vi "Spectrometer Triax 550 (N.O.).vi"(7 "Force Reset? (F)":bool, 8 "error in (no error)":errorcluster, 10 "Ref to a Status Box":refnum<vi>, 11 "Cluster In":T4) -> (0 "error out":errorcluster, 3 "Cluster Out":T4)   [LabVIEW 2009]
uses:
  JY-SPEX-TRIAX/controls.llb/Monochromator System Number.ctl
  JY-SPEX-TRIAX/controls.llb/Mirror Position.ctl
  JY-SPEX-TRIAX/controls.llb/Turret Position (TRIAX).ctl
  Global/GPIB Numbers.vi
  JY-SPEX-TRIAX/JY-SPEX-TRIAX.lvlib
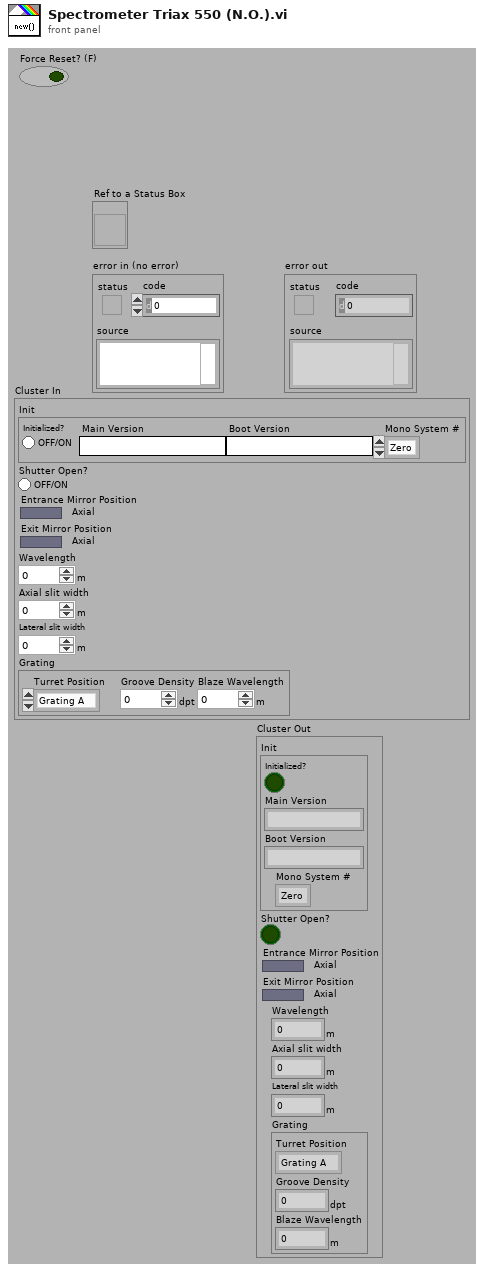
[diagram p1: front panel]
types:
  T1 = typedef "JY-SPEX-TRIAX.lvlib/Monochromator System Number.ctl" = enum16{"Zero", "One"}
  T2 = typedef "JY-SPEX-TRIAX.lvlib/Mirror Position.ctl" = bool
  T3 = typedef "JY-SPEX-TRIAX.lvlib/Turret Position (TRIAX).ctl" = enum16{"Grating A", "Grating B", "Grating C"}
  T4 = cluster{"Init":cluster{"Initialized?":bool, "Main Version":string, "Boot Version":string, "Mono System #":T1}, "Shutter Open?":bool, "Entrance Mirror Position":T2, "Exit Mirror Position":T2, "Wavelength":dbl[unit], "Axial slit width":dbl[unit], "Lateral slit width":dbl[unit], "Grating":cluster{"Turret Position":T3, "Groove Density":dbl[unit], "Blaze Wavelength":dbl[unit]}}
  T5 = typedef "GPIB Type Def.ctl" = cluster{"Name":string, "bus":dbl, "GPIB":dbl, "GPIB as string":string, "byte":i32, "VISA Resource Name":refnum<visa-resource-name>}
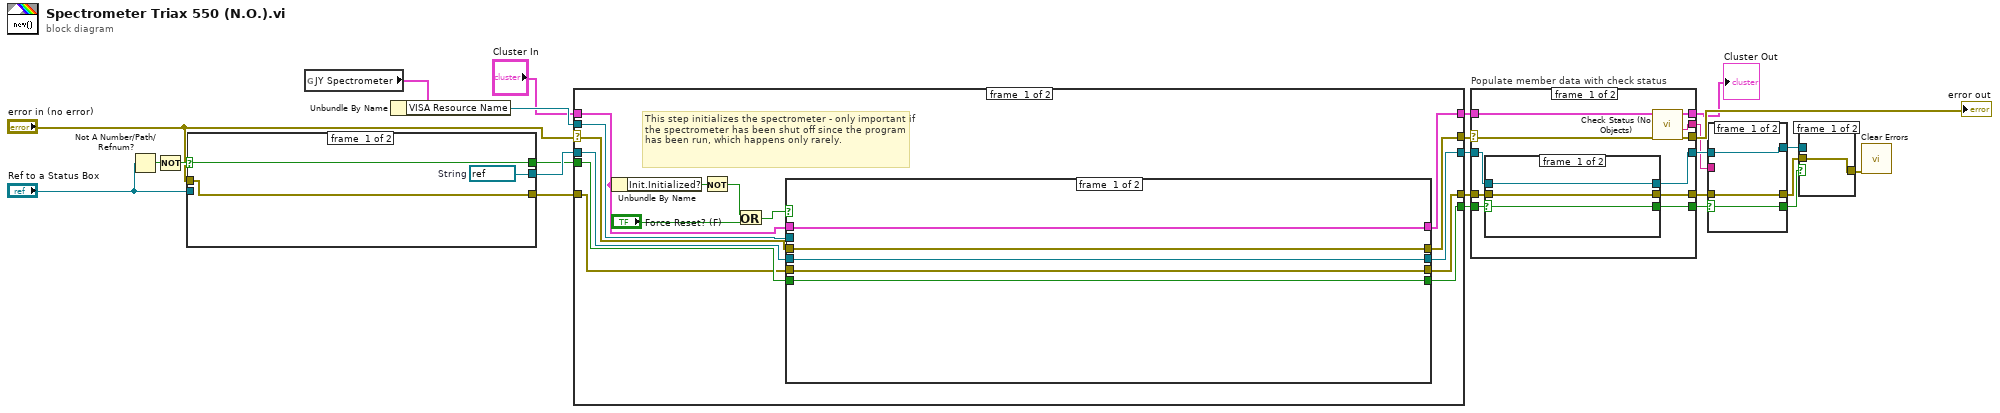
[diagram p0: block diagram]
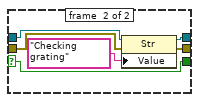
[diagram p2: hidden frame]
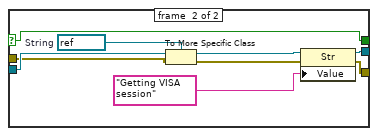
[diagram p4: hidden frame]
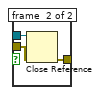
[diagram p5: hidden frame]
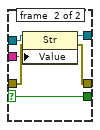
[diagram p6: hidden frame]
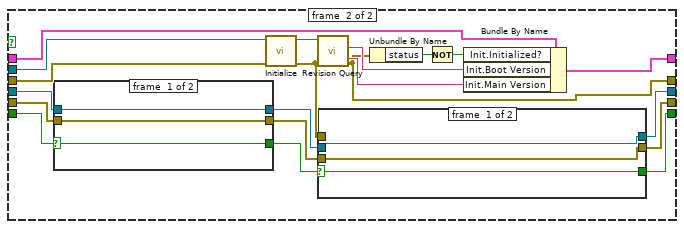
[diagram p7: hidden frame]
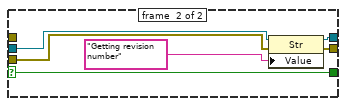
[diagram p8: hidden frame]
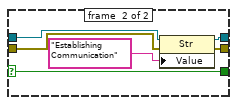
[diagram p9: hidden frame]
diagram:
  n1 = Not A Number/Path/Refnum?(number/path/refnum="Ref to a Status Box") -> (NaN/Path/Refnum?=w19:bool)
  n2 = Not(x=w19) -> (.not. x?=w7:bool)
  n3 = case shown="True" w7 {
    selector: w7 -> [w27 w34]
    tunnel: "error in (no error)" -> [w28 w29]
    tunnel: [w28 w37] -> w23
    tunnel: "Ref to a Status Box" -> [_ w32]
    tunnel: [w26 w35] -> w25
    tunnel: [w27 w34] -> w24
    frame #0 {
      w26 = refnum<vi> refnum  # String
    }
    frame #1 {
      w33 = refnum<vi> refnum  # String
      n4 = To More Specific Class(target class=w33, reference=w32, error in=w29) -> (specific class reference=w30:refnum<vi>, error out=w31:errorcluster)
      n5 = property class="Str"(reference=w30, error in=w31, "Value"="Getting VISA session") -> (reference out=w35:refnum<vi>, error out=w37:errorcluster)
    }
  }
  n6 = global read "GPIB Numbers.vi" "JY Spectrometer"() -> (w5:T5)
  n7 = Unbundle By Name(w5) -> ("VISA Resource Name"=w3:refnum<visa-resource-name>)
  n8 = case shown="No Error" "error in (no error)" {
    selector: "error in (no error)" -> [w43 w100]
    tunnel: [w46 w100] -> w6
    tunnel: "Cluster In" -> [w42 w99]
    tunnel: w3 -> [w52 _]
    tunnel: [w51 w99] -> w18
    tunnel: w25 -> [w50 w98]
    tunnel: [w47 w98] -> w16
    tunnel: w24 -> [w49 w97]
    tunnel: [w48 w97] -> w14
    tunnel: w23 -> [w45 w96]
    tunnel: [w44 w96] -> w11
    frame #0 {
      # "This step initializes the spectrometer - only important if the spectrometer has been shut off since the program has been run, which happens only rarely."
      n9 = Unbundle By Name(w42) -> ("Init.Initialized?"=w40:bool)
      n10 = Not(x=w40) -> (.not. x?=w41:bool)
      n11 = Or(x=w41, y="Force Reset? (F)") -> (x .or. y?=w38:bool)
      n12 = case shown="True" w38 {
        tunnel: w42 -> [w57 w73]
        tunnel: w52 -> [_ w72]
        tunnel: [w57 w59] -> w51
        tunnel: w50 -> [w55 w71]
        tunnel: w49 -> [w53 w70]
        tunnel: [w53 w68] -> w48
        tunnel: [w55 w66] -> w47
        tunnel: [w56 w58] -> w46
        tunnel: w45 -> [w54 w65]
        tunnel: [w54 w63] -> w44
        tunnel: w43 -> [w56 w62]
        frame #0 {
        }
        frame #1 {
          n13 = case shown="True" w70 {
            selector: w70 -> [w87 w90]
            tunnel: w65 -> [w88 w95]
            tunnel: [w88 w94] -> w64
            tunnel: w71 -> [w89 w93]
            tunnel: [w89 w91] -> w67
            tunnel: [w87 w90] -> w69
            frame #0 {
            }
            frame #1 {
              n14 = property class="Str"(reference=w93, error in=w95, "Value"="Establishing Communication") -> (reference out=w91:refnum<vi>, error out=w94:errorcluster)
            }
          }
          n15 = call "Initialize.vi"("error in (no error)"=w62, "VISA resource name"=w72) -> ("error out"=w60:errorcluster, "VISA resource name out"=w77:refnum<visa-resource-name>)  [unwired: 8 out]
          n16 = call "Revision Query.vi"("error in (no error)"=w60, "VISA resource name"=w77) -> ("error out"=w58:errorcluster, "Main Firmware Revision"=w74:string, "Boot Firmware Revision"=w75:string)  [unwired: 7 out]
          n17 = case shown="True" w69 {
            selector: w69 -> [w78 w81]
            tunnel: w64 -> [w79 w86]
            tunnel: [w79 w85] -> w63
            tunnel: w67 -> [w80 w84]
            tunnel: [w80 w82] -> w66
            tunnel: [w78 w81] -> w68
            tunnel: w60 -> [_ _]
            frame #0 {
            }
            frame #1 {
              n18 = property class="Str"(reference=w84, error in=w86, "Value"="Getting revision number") -> (reference out=w82:refnum<vi>, error out=w85:errorcluster)
            }
          }
          n19 = Unbundle By Name(w58) -> ("status"=w76:bool)
          n20 = Not(x=w76) -> (.not. x?=w61:bool)
          n21 = Bundle By Name(cluster=w73, "Init.Initialized?"=w61, "Init.Boot Version"=w75, "Init.Main Version"=w74) -> (w59:T4)
        }
      }
    }
    frame #1 {
    }
  }
  n22 = case "Populate member data with check status" shown="No Error" w6 {
    selector: w6 -> [w102 w124]
    tunnel: w18 -> [w101 w125]
    tunnel: [w111 w124] -> w17
    tunnel: [w110 w125] -> w1
    tunnel: w16 -> [w109 w122]
    tunnel: [w108 w122] -> w15
    tunnel: w14 -> [w107 w123]
    tunnel: [w106 w123] -> w13
    tunnel: [w105 w121] -> w12
    tunnel: w11 -> [w104 w121]
    tunnel: [w103 _] -> w10
    frame #0 {
      n23 = case shown="True" w107 {
        selector: w107 -> [w114 w118]
        tunnel: [w112 w120] -> w105
        tunnel: [w114 w118] -> w106
        tunnel: [w113 w117] -> w108
        tunnel: w104 -> [w112 w116]
        tunnel: w109 -> [w113 w115]
        frame #0 {
        }
        frame #1 {
          n24 = property class="Str"(reference=w115, error in=w116, "Value"="Checking grating") -> (reference out=w117:refnum<vi>, error out=w120:errorcluster)
        }
      }
      n25 = call "Check Status (No Objects).vi"("error in (no error)"=w102, "Cluster In"=w101) -> ("error out"=w111:errorcluster, "Status"=w103:string, "Cluster Out"=w110:T4)  [unwired: 6 in, 1 out]
    }
    frame #1 {
    }
  }
  "error out" <- w17
  "Cluster Out" <- w1
  n26 = case shown="True" w13 {
    selector: w13 -> [w128 w132]
    tunnel: [w127 w134] -> w22
    tunnel: [w126 w133] -> w9
    tunnel: [w128 w132] -> w8
    tunnel: w15 -> [w126 w131]
    tunnel: w12 -> [w127 w130]
    tunnel: w10 -> [_ w129]
    frame #0 {
    }
    frame #1 {
      n27 = property class="Str"(reference=w131, error in=w130, "Value"=w129) -> (reference out=w133:refnum<vi>, error out=w134:errorcluster)
    }
  }
  n28 = case shown="True" w8 {
    tunnel: w22 -> [w135 w138]
    tunnel: [w135 w137] -> w21
    tunnel: w9 -> [_ w136]
    frame #0 {
    }
    frame #1 {
      n29 = Close Reference(reference=w136, error in (no error)=w138) -> (error out=w137:errorcluster)
    }
  }
  n30 = call <vilib>:"Clear Errors.vi"("error in (no error)"=w21) -> ()  [unwired: 7 out]
